vi "ExtImgFGV.vi"(7 "Enum":enum16{"set", "read", "close"}(ring), 8 "error in":errorcluster, 11 "Image In":T1(plugin-control)) -> (0 "error out":errorcluster, 3 "Image Out":T1(plugin-control))   [LabVIEW 2018]
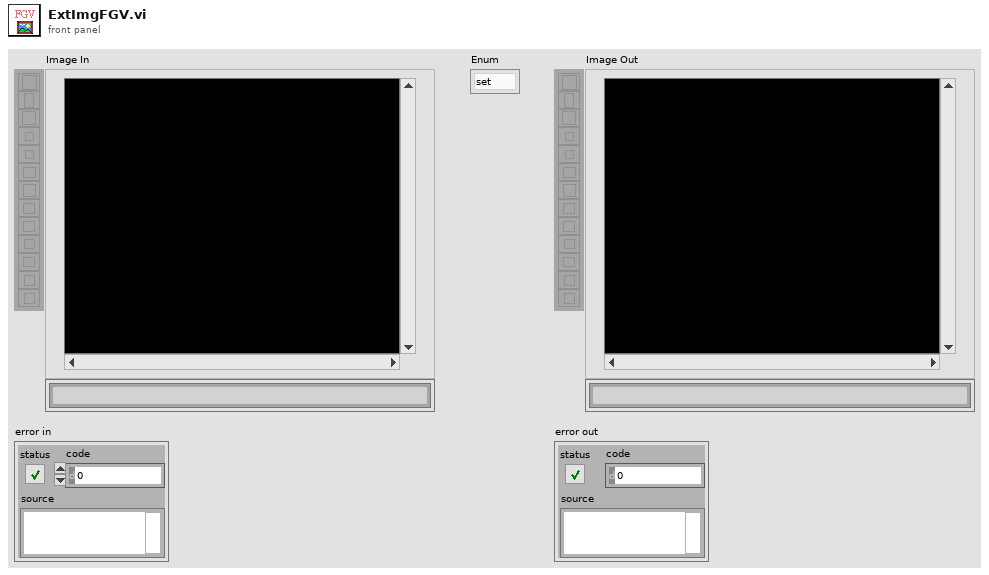
[diagram p1: front panel]
types:
  T1 = typedef "IMAQ Image.ctl" = refnum<image>
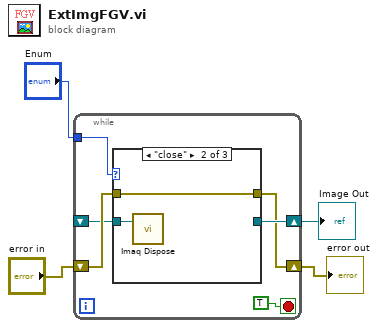
[diagram p0: block diagram]
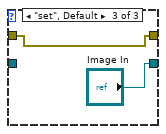
[diagram p3: hidden frame]
diagram:
  n1 = while {
    tunnel: "Enum" -> [w8]
    shift-right: [w5] -> w3
    shift-left: "error in" -> [w9]
    shift-right: [w7] -> w1
    shift-left: _ -> [w6]
    stop <- TRUE stop-if-true
    n2 = case shown="\"close\"" w8 {
      tunnel: [w12 w14 w16] -> w5
      tunnel: w9 -> [w12 w14 w16]
      tunnel: [w11 _ "Image In"] -> w7
      tunnel: w6 -> [w11 w13 _]
      frame "read" {
      }
      frame "close" {
        n3 = call "Imaq Dispose"("Image"=w13) -> ()  [unwired: 5 in, 1 out]
      }
      frame "set", Default {
      }
    }
  }
  "Image Out" <- w1
  "error out" <- w3
